vi "Get VISA Resource.vi"(8 "error in (no error)":errorcluster, 11 "niDTS Comm Serial in":refnum<class "niDTS Comm Serial.lvclass">) -> (0 "error out":errorcluster, 2 "VISA Resource":refnum<visa-resource-name>="COM1", 3 "niDTS Comm Serial out":refnum<class "niDTS Comm Serial.lvclass">)   [LabVIEW 2015, in "niDTS CommLib.lvlib" / "niDTS Comm Serial.lvclass"]
uses:
  niDTS Comm Serial.lvclass
  niDTS Comm Serial.lvclass/niDTS Comm Serial.ctl
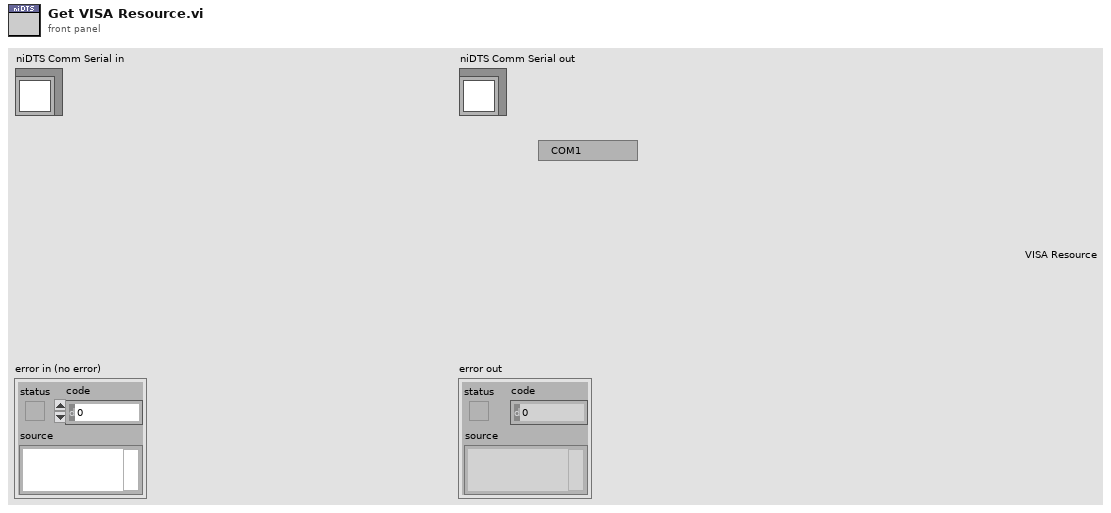
[diagram p1: front panel]
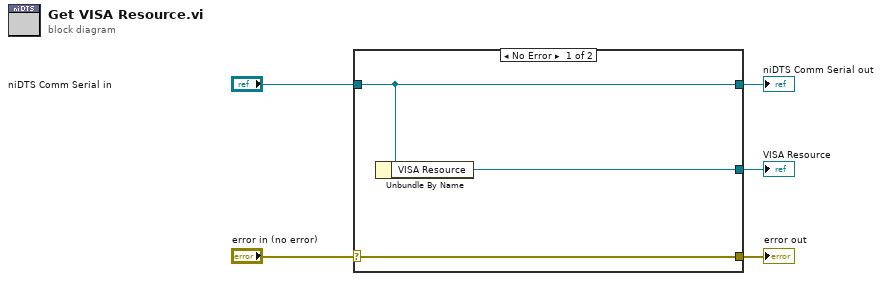
[diagram p0: block diagram]
diagram:
  n1 = case shown="No Error" "error in (no error)" {
    selector: "error in (no error)" -> [w8 w9]
    tunnel: [w8 w9] -> w4
    tunnel: [w7 w10] -> w2
    tunnel: "niDTS Comm Serial in" -> [w7 w10]
    tunnel: [w6 _] -> w1
    frame No Error {
      n2 = Unbundle By Name(w7) -> ("VISA Resource"=w6:refnum<visa-resource-name>)
    }
    frame Error {
    }
  }
  "error out" <- w4
  "niDTS Comm Serial out" <- w2
  "VISA Resource" <- w1
